vi "data insert.vi"(8 "error in (no error)":errorcluster, 10 "data in":T1={"水样数据时间"=timestamp(0 s since 1904-01-01), "测量模式"="", "数据类型"="N", "水样实测值"=0.0, "单位"="", "水样数据标识"="N", "信号值"=0.0, "标样参考值"=0.0, "因子编码"="", "探头温度"=0.0}, 11 "table in":string(combo)) -> (0 "error out":errorcluster)   [LabVIEW 2016, in "斯坦道多参数.lvlib"]
uses:
  <vilib>/addons/database/Auxilliary.llb/DB Tools Column Info.ctl
  <vilib>/addons/database/Auxilliary.llb/DB Tools DataTypes.ctl
  <vilib>/addons/database/NI_Database_API.lvlib
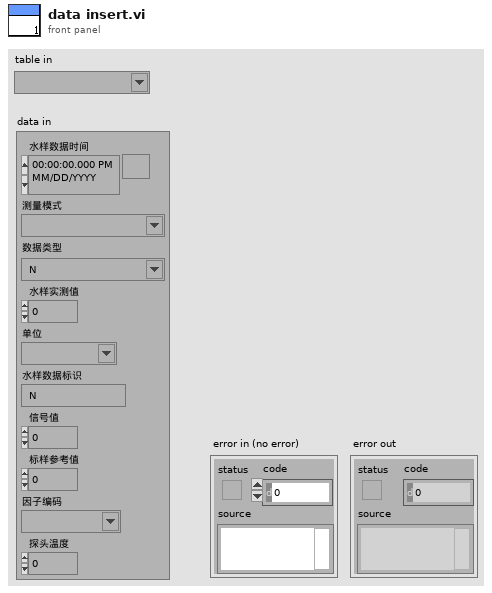
[diagram p1: front panel]
types:
  T1 = cluster{"水样数据时间":timestamp, "测量模式":string, "数据类型":string, "水样实测值":sgl, "单位":string, "水样数据标识":string, "信号值":sgl, "标样参考值":sgl, "因子编码":string, "探头温度":sgl}
  T2 = typedef "NI_Database_API.lvlib/DB Tools Column Info.ctl" = cluster{"column name":string, "data type":T3, "size":i32, "allow null?":bool}
  T3 = typedef "NI_Database_API.lvlib/DB Tools DataTypes.ctl" = enum16{"String", "Long (I32)", "Single (SGL)", "Double (DBL)", "Date/Time", "Binary"}
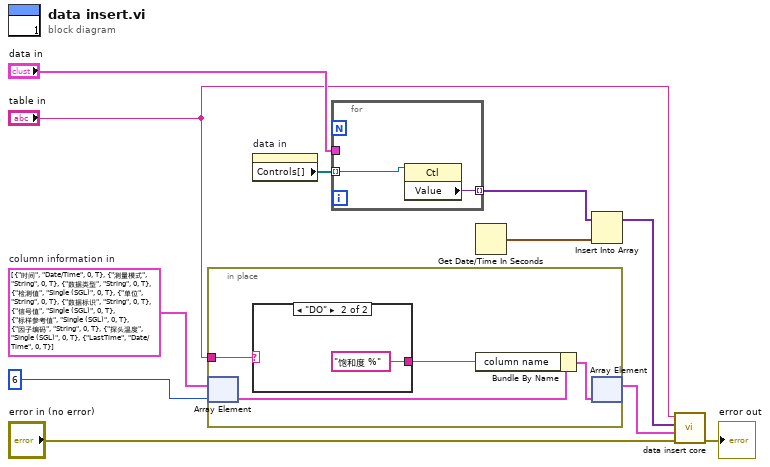
[diagram p0: block diagram]
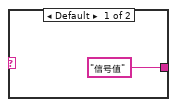
[diagram p2: hidden frame]
diagram:
  w2 = T2[] [{"column name"="时间", "data type"=enum."Date/Time", "size"=0, "allow null?"=TRUE}, {"column name"="测量模式", "data type"=enum."String", "size"=0, "allow null?"=TRUE}, {"column name"="数据类型", "data type"=enum."String", "size"=0, "allow null?"=TRUE}, {"column name"="检测值", "data type"=enum."Single (SGL)", "size"=0, "allow null?"=TRUE}, {"column name"="单位", "data type"=enum."String", "size"=0, "allow null?"=TRUE}, {"column name"="数据标识", "data type"=enum."String", "size"=0, "allow null?"=TRUE}, {"column name"="信号值", "data type"=enum."Single (SGL)", "size"=0, "allow null?"=TRUE}, {"column name"="标样参考值", "data type"=enum."Single (SGL)", "size"=0, "allow null?"=TRUE}, {"column name"="因子编码", "data type"=enum."String", "size"=0, "allow null?"=TRUE}, {"column name"="探头温度", "data type"=enum."Single (SGL)", "size"=0, "allow null?"=TRUE}, {"column name"="LastTime", "data type"=enum."Date/Time", "size"=0, "allow null?"=TRUE}]  # column information in
  n1 = in-place {
    in-place-border: "table in" -> [w15]
    n2 = in-place-array #1(w2, 6) -> (w12:T2)
    n3 = case shown="\"DO\"" w15 {
      tunnel: ["信号值" ("column name") "饱和度 %" ("column name")] -> w14
      frame Default {
      }
      frame "DO" {
      }
    }
    n4 = Bundle By Name(cluster=w12, "column name"=w14) -> (w13:T2)
    n5 = in-place-array #1(w13) -> (w1:T2[])  [unwired: 1 out]
  }
  n6 = property on="data in" class="Clust (严格)"() -> ("Controls[]"=w11:refnum<vi>[])  [unwired: 2 in, 2 out]
  n7 = for {
    tunnel: w11 -> [w19] mode=indexing
    tunnel: [w18] -> w9 mode=indexing
    tunnel: "data in" -> [_]
    n8 = property class="Ctl"(reference=w19) -> ("Value"=w18:variant)  [unwired: 1 in, 2 out]
  }
  n9 = Get Date/Time In Seconds() -> (seconds since 1Jan1904=w8:timestamp)
  n10 = Insert Into Array(array=w9, new element=w8) -> (w7:variant[])  [unwired: 1 in]
  n11 = call "data insert core.vi"("error in (no error)"="error in (no error)", "column information"=w1, "data"=w7, "table"="table in") -> ("error out"=→"error out":errorcluster)  [unwired: 7 in]
